vi "Scrub Variants.vi"(11 "Graph In":T1[](array[typedef])) -> (3 "Cleaned Graph":T1[](array[typedef]))   [LabVIEW 2020, in "Better Search.lvlib"]
uses:
  Better Search.lvlib
  Data Types/Type Reflection Item.ctl
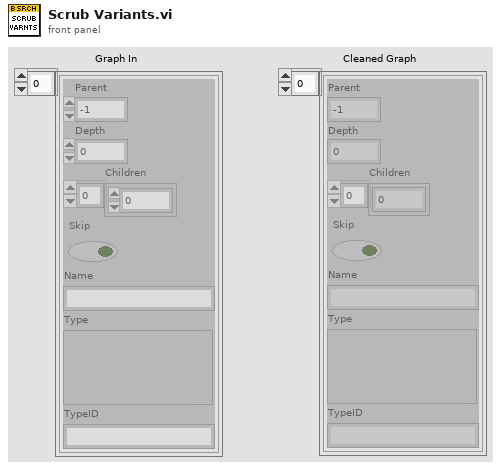
[diagram p1: front panel]
types:
  T1 = typedef "Better Search.lvlib/Type Reflection Item.ctl" = cluster{"Parent":i32, "Depth":i32, "Children":i32[], "Skip":bool, "Name":string, "Type":variant, "TypeID":string}
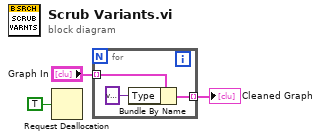
[diagram p0: block diagram]
diagram:
  n1 = Request Deallocation(TRUE ("flag")) -> ()
  n2 = for {
    tunnel: "Graph In" -> [w6] mode=indexing
    tunnel: [w4] -> w1 mode=indexing
    n3 = Bundle By Name(cluster=w6, "Type"=variant) -> (w4:T1)
  }
  "Cleaned Graph" <- w1
